vi "Practica 03.vi"() -> ()   [LabVIEW 2011]
panel:
  in  "PUERTO SERIAL":refnum<visa-resource-name>
  in  "stop":bool
  in  "OK Button 2":bool
  in  "[PA:13]":dbl=1.0
  in  "[PA:12]":dbl=1.0
  in  "Velocidad (PTO)":u32=60000
  out "Alarma !":bool
  in  "Posicion (mm)":dbl(slide) scale=0.0..750.0
  in  "OK Button":bool
  in  "SERVO ON":bool
  # "Deslizador Lineal UTN"
  # "CONTOL DE POSICIÓN"
  # "CONTROL DE POSICIÓN - Lazo abierto"
  # "1. Encender el servomotor"
  # "2. Escojer Posición"
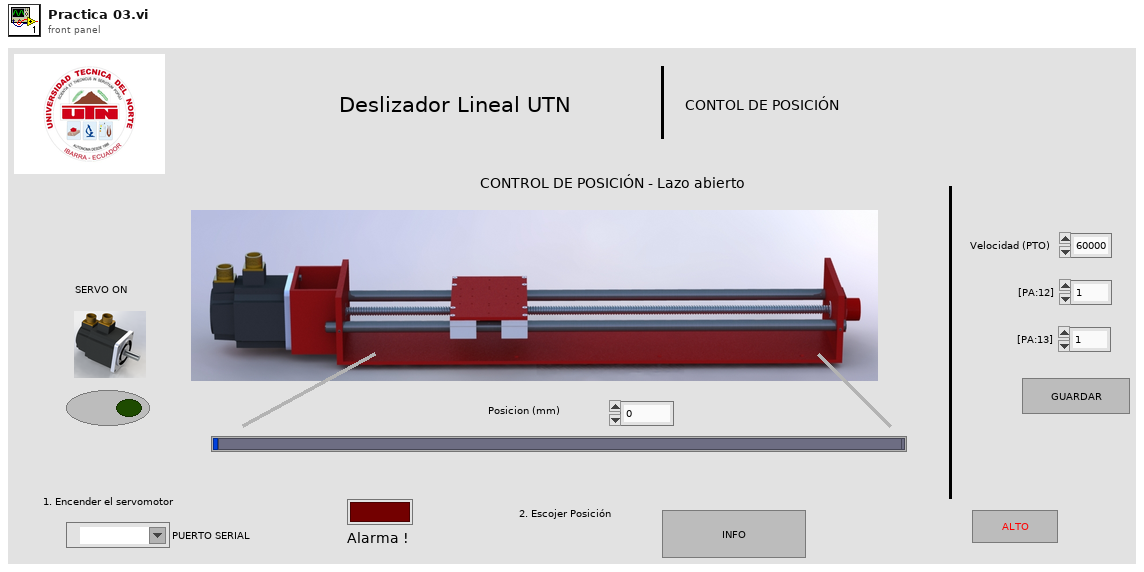
[diagram p1: front panel]
types:
  T1 = enum16{"Aout", "Fout", "Direccion", "ServoOn", "Idle"}
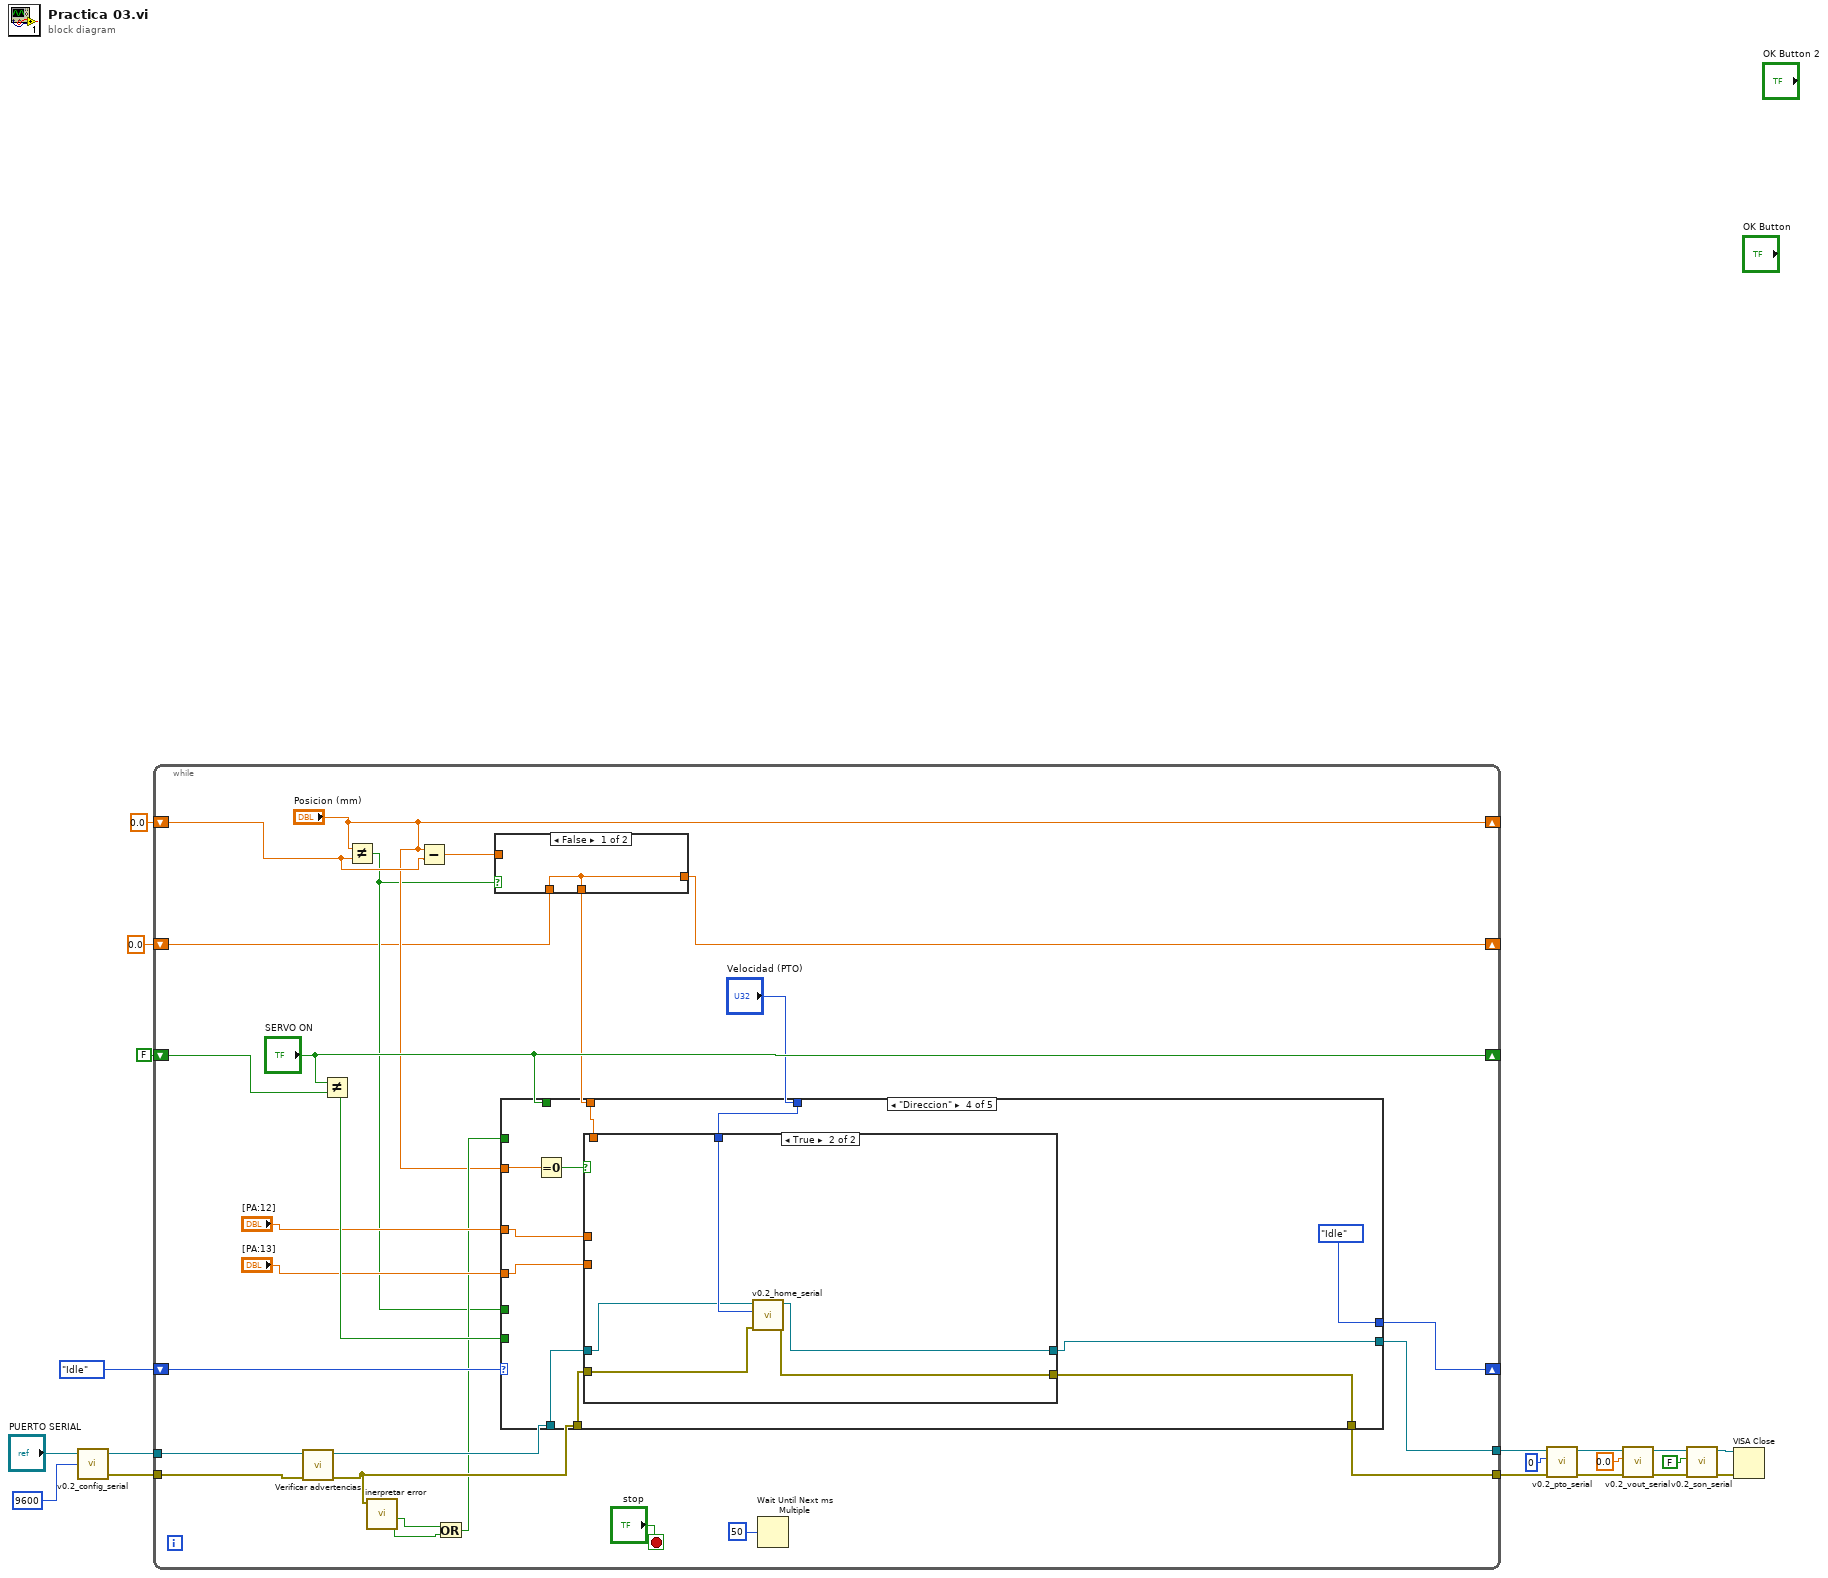
[diagram p0: block diagram]
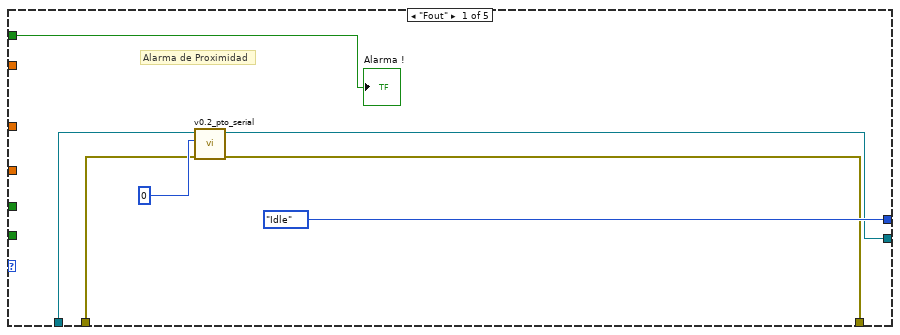
[diagram p3: hidden frame]
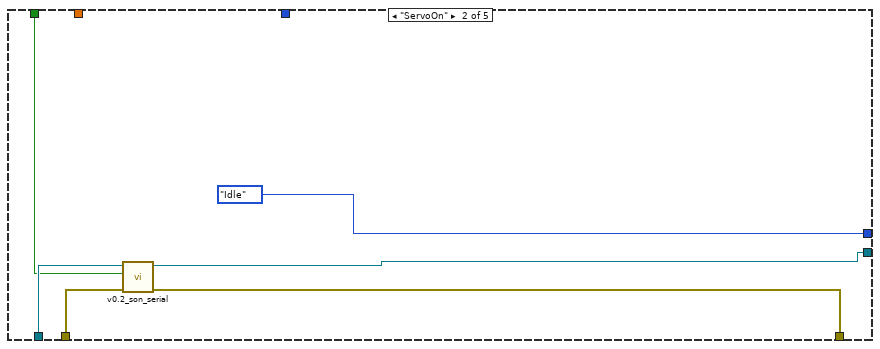
[diagram p4: hidden frame]
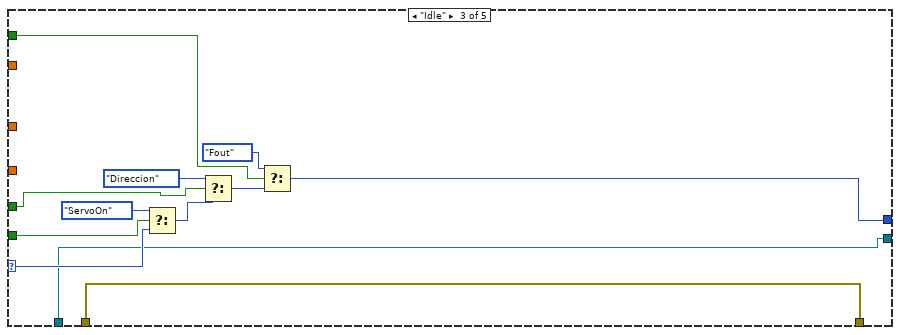
[diagram p5: hidden frame]
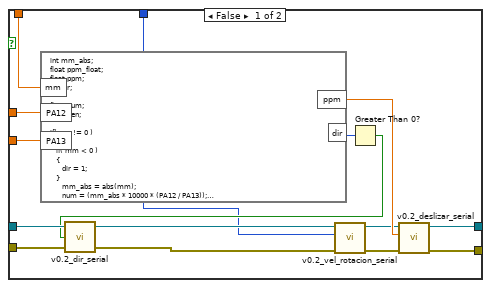
[diagram p6: hidden frame]
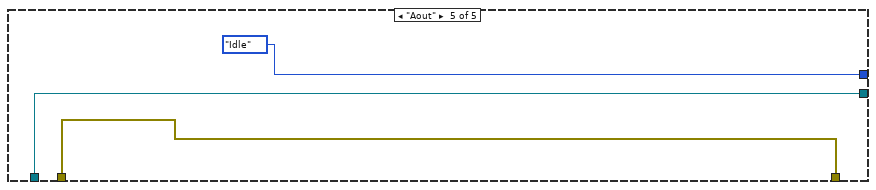
[diagram p7: hidden frame]
diagram:
  n1 = call "v0.2_config_serial.vi"("baud rate (9600/115200)"=u32 9600, "VISA COM IN"="PUERTO SERIAL") -> ("error out"=w17:errorcluster, "VISA COM OUT"=w18:refnum<visa-resource-name>)  [unwired: 2 in]
  n2 = while {
    tunnel: w18 -> [w38]
    tunnel: w17 -> [w37]
    tunnel: [w39] -> w10
    shift-right: [w42] -> _
    shift-left: T1."Idle" -> [w43]
    shift-right: ["Posicion (mm)"] -> _
    shift-left: 0.0 ("Posicion (mm)") -> [w27]
    shift-right: ["SERVO ON"] -> _
    shift-left: FALSE ("SON") -> [w41]
    tunnel: [w25] -> w14
    shift-right: [w21] -> _
    shift-left: 0.0 -> [w20]
    stop <- "stop" stop-if-true
    n3 = call "Verificar advertencias.vi"("error in"=w37, "VISA COM IN"=w38) -> ("error out"=w35:errorcluster, "VISA COM OUT"=w36:refnum<visa-resource-name>)  [unwired: 8 in]
    n4 = Not Equal?(x="SERVO ON", y=w41) -> (x != y?=w40:bool)
    n5 = Not Equal?(x="Posicion (mm)", y=w27) -> (x != y?=w24:bool)
    n6 = call "inerpretar error.vi"("error out"=w35) -> ("Alarma Proximidad Encoder"=w33:bool, "Alarma Proximidad MOtor"=w34:bool)  [unwired: 5 in, 4 out]
    n7 = Subtract(x="Posicion (mm)", y=w27) -> (x-y=w23:dbl)
    n8 = Or(x=w34, y=w33) -> (x .or. y?=w28:bool)
    n9 = case shown="False" w24 {
      tunnel: w23 -> [_ w47]
      tunnel: [w46 w47] -> w22
      tunnel: [w46 w47] -> w21
      tunnel: w20 -> [w46 _]
      frame False {
      }
      frame True {
      }
    }
    n10 = case shown="\"Direccion\"" w43 {
      selector: w43 -> [_ _ w66 _ _]
      tunnel: w28 -> [w49 _ w72 _ _]
      tunnel: [T1."Idle" T1."Idle" w70 T1."Idle" T1."Idle"] -> w42
      tunnel: w24 -> [_ _ w64 _ _]
      tunnel: w40 -> [_ _ w65 _ _]
      tunnel: w36 -> [w52 w60 w61 w82 w104]
      tunnel: "Velocidad (PTO)" -> [_ _ _ w77 _]
      tunnel: "SERVO ON" -> [_ w59 _ _ _]
      tunnel: w35 -> [w51 w57 w63 w81 w106]
      tunnel: [w50 w56 w63 w74 w106] -> w39
      tunnel: "[PA:12]" -> [_ _ _ w80 _]
      tunnel: "[PA:13]" -> [_ _ _ w79 _]
      tunnel: "Posicion (mm)" -> [_ _ _ w78 _]
      tunnel: [w48 w55 w61 w75 w104] -> w25
      tunnel: w22 -> [_ _ _ w76 _]
      frame "Fout" {
        # "Alarma de Proximidad"
        n11 = call "v0.2_pto_serial.vi"("error in (no error)"=w51, "Fout"=u32 0, "VISA COM IN"=w52) -> ("error out"=w50:errorcluster, "VISA COM OUT"=w48:refnum<visa-resource-name>)  [unwired: 7 in]
        "Alarma !" <- w49
      }
      frame "ServoOn" {
        n12 = call "v0.2_son_serial.vi"("error in (no error)"=w57, "ServoON"=w59, "VISA COM IN"=w60) -> ("error out"=w56:errorcluster, "VISA COM OUT"=w55:refnum<visa-resource-name>)  [unwired: 7 in]
      }
      frame "Idle" {
        n13 = Select(t=T1."ServoOn", s=w65, f=w66) -> (s? t:f=w67:T1)
        n14 = Select(t=T1."Direccion", s=w64, f=w67) -> (s? t:f=w62:T1)
        n15 = Select(t=T1."Fout", s=w72, f=w62) -> (s? t:f=w70:T1)
      }
      frame "Direccion" {
        n16 = Equal To 0?(x=w78) -> (x = 0?=w73:bool)
        n17 = case shown="True" w73 {
          tunnel: w82 -> [w98 w102]
          tunnel: w81 -> [w97 w100]
          tunnel: w80 -> [w96 _]
          tunnel: w79 -> [w95 _]
          tunnel: [w91 w101] -> w75
          tunnel: [w90 w99] -> w74
          tunnel: w77 -> [w85 w103]
          tunnel: w76 -> [w84 _]
          frame False {
            n18 = formula code="int mm_abs;\nfloat ppm_float;\nfloat ppm;\nint dir;\n\nfloat num;\nfloat den;\n\nif(mm != 0 )\n{\n   if( mm < 0 )\n   {\n      dir = 1;\n   }\n      mm_abs = abs(mm);\n      num = (mm_abs * 10000 * (PA12 / PA13));\n      den = 5 * 1000;\n      ppm = num / den;\n}"("PA12"=w96, "PA13"=w95, "mm"=w84) -> ("ppm"=w92:dbl, "dir"=w94:i32)
            n19 = Greater Than 0?(x=w94) -> (x > 0?=w93:bool)
            n20 = call "v0.2_dir_serial.vi"("error in (no error)"=w97, "Direccion"=w93, "VISA COM IN"=w98) -> ("error out"=w87:errorcluster, "VISA COM OUT"=w89:refnum<visa-resource-name>)  [unwired: 1 in]
            n21 = call "v0.2_vel_rotacion_serial.vi"("error in (no error)"=w87, "RPM's Rotacion"=w85, "VISA COM IN"=w89) -> ("error out"=w86:errorcluster, "VISA COM OUT"=w88:refnum<visa-resource-name>)  [unwired: 7 in]
            n22 = call "v0.2_deslizar_serial.vi"("error in (no error)"=w86, "Fout"=w92, "VISA COM IN"=w88) -> ("error out"=w90:errorcluster, "VISA COM OUT"=w91:refnum<visa-resource-name>)  [unwired: 7 in]
          }
          frame True {
            n23 = call "v0.2_home_serial.vi"("error in (no error)"=w100, "Fout"=w103, "VISA COM IN"=w102) -> ("error out"=w99:errorcluster, "VISA COM OUT"=w101:refnum<visa-resource-name>)  [unwired: 7 in]
          }
        }
      }
      frame "Aout" {
      }
    }
    n24 = Wait Until Next ms Multiple(millisecond multiple=u32 50) -> ()  [unwired: 1 out]
  }
  n25 = call "v0.2_pto_serial.vi"("error in (no error)"=w10, "Fout"=u32 0, "VISA COM IN"=w14) -> ("error out"=w9:errorcluster, "VISA COM OUT"=w13:refnum<visa-resource-name>)  [unwired: 7 in]
  n26 = call "v0.2_vout_serial.vi"("error in (no error)"=w9, "Volt"=0.0, "VISA COM IN"=w13) -> ("error out"=w8:errorcluster, "VISA COM OUT"=w12:refnum<visa-resource-name>)  [unwired: 7 in]
  n27 = call "v0.2_son_serial.vi"("error in (no error)"=w8, "ServoON"=FALSE, "VISA COM IN"=w12) -> ("error out"=w7:errorcluster, "VISA COM OUT"=w11:refnum<visa-resource-name>)  [unwired: 7 in]
  n28 = VISA Close(VISA resource name=w11, error in (no error)=w7) -> ()  [unwired: 1 out]
